vi "Tosca-Baseline Dialog.vi"(7 "milliseconds to wait":u32) -> (8 "aborted?":bool)   [LabVIEW 2020]
panel:
  in  "Skip Button":bool
  in  "Abort Button":bool
  # "Baseline period..."
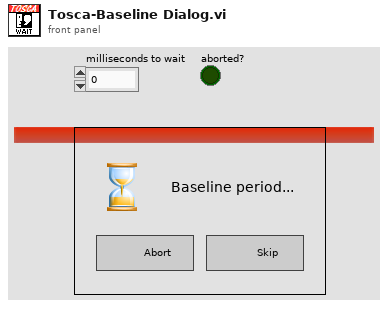
[diagram p1: front panel]
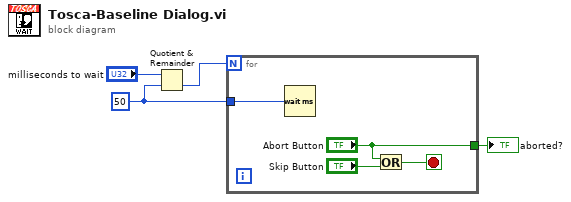
[diagram p0: block diagram]
diagram:
  w2 = u32 50 ("y")
  n1 = Quotient & Remainder(x="milliseconds to wait", y=w2) -> (floor(x/y)=w1:u32)  [unwired: 1 out]
  n2 = for {
    N: w1 -> [_]
    tunnel: ["Abort Button"] -> w4
    tunnel: w2 -> [w5]
    stop <- w6 stop-if-true
    n3 = Wait (ms)(milliseconds to wait=w5) -> ()  [unwired: 1 out]
    n4 = Or(x="Abort Button", y="Skip Button") -> (x .or. y?=w6:bool)
  }
  "aborted?" <- w4
